vi "Initiate.vi"(8 "error in (no error)":errorcluster, 10 "Initiate Type (0: Immediate)":i32(ring) items=["Immediate", "Continuous"], 11 "VISA resource name":refnum<visa-resource-name>) -> (0 "error out":errorcluster, 3 "VISA resource name out":refnum<visa-resource-name>)   [LabVIEW 2025, in "Keithley 2182.lvlib"]
doc: "Initiates one or continuous trigger cycle(s).\n\n<B>Note:</B>\nTo disable continuous initiation, set the instrument to Immediate Initiation."
uses:
  Keithley 2182.lvlib
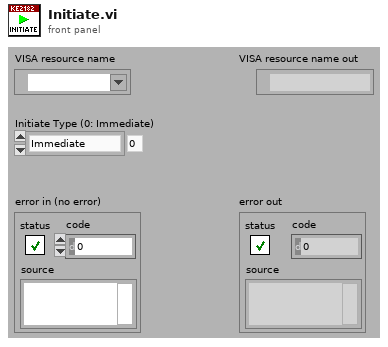
[diagram p1: front panel]
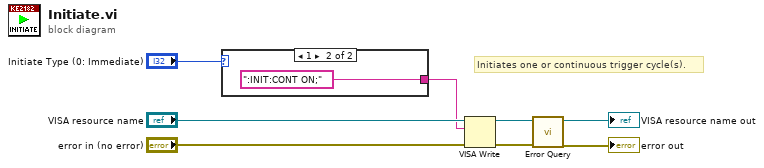
[diagram p0: block diagram]
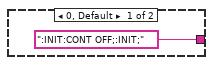
[diagram p2: hidden frame]
diagram:
  # "Initiates one or continuous trigger cycle(s)."
  n1 = case shown="1" "Initiate Type (0: Immediate)" {
    tunnel: [":INIT:CONT OFF;:INIT;" ":INIT:CONT ON;"] -> w1
    frame 0, Default {
    }
    frame 1 {
    }
  }
  n2 = VISA Write(VISA resource name="VISA resource name", write buffer=w1, error in (no error)="error in (no error)") -> (VISA resource name out=w6:refnum<visa-resource-name>, error out=w5:errorcluster)  [unwired: 1 out]
  n3 = call "Error Query.vi"("error in (no error)"=w5, "VISA resource name"=w6) -> ("error out"=→"error out":errorcluster, "VISA resource name out"=→"VISA resource name out":refnum<visa-resource-name>)  [unwired: 6 in, 2 out]
